vi "Get Data.vi"(8 "error in (no error)":errorcluster, 11 "DataGrid.lvlib:Abstract EVENT.lvclass":refnum<class "Abstract EVENT.lvclass">) -> (0 "error out":errorcluster, 2 "output cluster":T1)   [LabVIEW 2013, in "DataGrid.lvlib" / "KeyDown.lvclass"]
doc: "Converts the class data for key down into individual components of the grid"
uses:
  KeyDown.lvclass
  Abstract EVENT/Abstract EVENT.lvclass
  KeyDown.lvclass/KeyDown.ctl
  Read Alt.vi
  Read Control.vi
  Read KeyCode.vi
  Read KeyData.vi
  Read KeyValue.vi
  Read Modifiers.vi
  Read Shift.vi
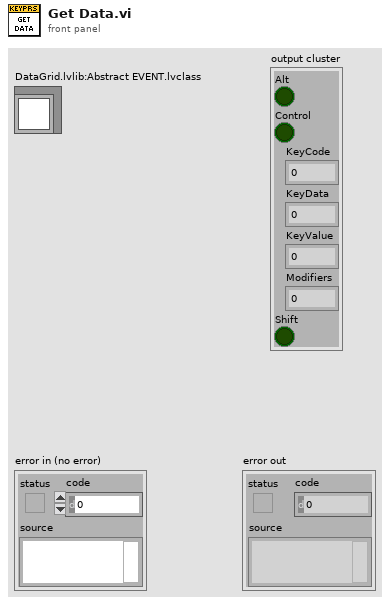
[diagram p1: front panel]
types:
  T1 = cluster{"Alt":bool, "Control":bool, "KeyCode":i32, "KeyData":i32, "KeyValue":i32, "Modifiers":i32, "Shift":bool}
  T2 = cluster{"Properties:Alt":bool, "Properties:Control":bool, "Properties:KeyCode":i32, "Properties:KeyData":i32, "Properties:KeyValue":i32, "Properties:Modifiers":i32, "Properties:Shift":bool}
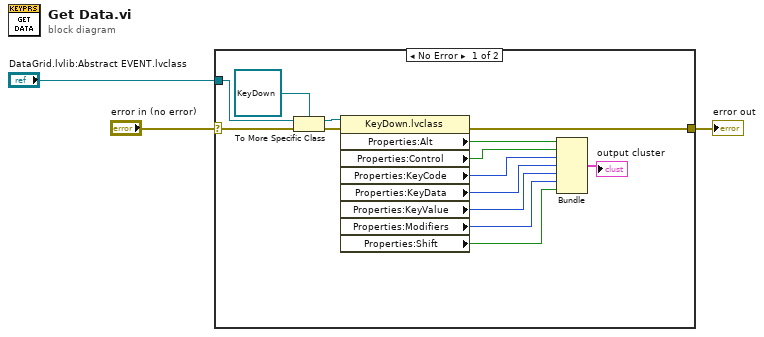
[diagram p0: block diagram]
diagram:
  n1 = case shown="No Error" "error in (no error)" {
    selector: "error in (no error)" -> [w13 w18]
    tunnel: [w17 w18] -> w2
    tunnel: "DataGrid.lvlib:Abstract EVENT.lvclass" -> [w15 _]
    frame No Error {
      n2 = To More Specific Class(target class=refnum<class "KeyDown.lvclass"> refnum ("DataGrid.lvlib:CellValueChanged.lvclass"), reference=w15, error in=w13) -> (specific class reference=w14:refnum<class "KeyDown.lvclass">, error out=w12:errorcluster)
      n3 = property class="KeyDown.lvclass"(reference=w14, error in=w12) -> (error out=w17:errorcluster, "Properties:Alt"=w11:bool, "Properties:Control"=w10:bool, "Properties:KeyCode"=w9:i32, "Properties:KeyData"=w8:i32, "Properties:KeyValue"=w7:i32, "Properties:Modifiers"=w6:i32, "Properties:Shift"=w5:bool)  [unwired: 1 out]
      n4 = Bundle("Properties:Alt"=w11, "Properties:Control"=w10, "Properties:KeyCode"=w9, "Properties:KeyData"=w8, "Properties:KeyValue"=w7, "Properties:Modifiers"=w6, "Properties:Shift"=w5) -> (→"output cluster":T2)  [unwired: 1 in]
    }
    frame Error {
    }
  }
  "error out" <- w2
